vi "Read Voltage From Channel.vi"(8 "error in (no error)":errorcluster, 10 "Numeric":u8, 11 "IConfigure MultiChannel Voltmeter in":refnum<class "IConfigure MultiChannel Voltmeter.lvclass">) -> (0 "error out":errorcluster, 2 "Voltage":dbl format="%#_g V", 3 "IConfigure MultiChannel Voltmeter out":refnum<class "IConfigure MultiChannel Voltmeter.lvclass">)   [LabVIEW 2023, in "HAL Interfaces.lvlib" / "IConfigure MultiChannel Voltmeter.lvclass"]
uses:
  IConfigure MultiChannel Voltmeter.lvclass
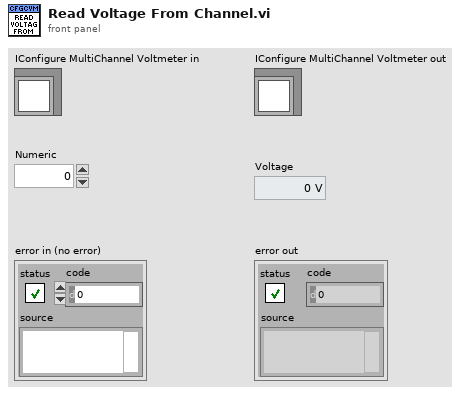
[diagram p1: front panel]
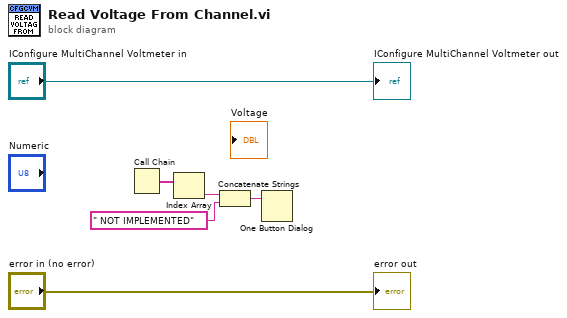
[diagram p0: block diagram]
diagram:
  n1 = Call Chain() -> (call chain=w4:string[])
  n2 = Index Array(array=w4) -> (element=w2:string)  [unwired: 1 in]
  n3 = Concatenate Strings(w2, " NOT IMPLEMENTED" ("string")) -> (w3:string)
  n4 = One Button Dialog(message=w3) -> ()  [unwired: 1 in, 1 out]
  "error out" <- "error in (no error)"
  "IConfigure MultiChannel Voltmeter out" <- "IConfigure MultiChannel Voltmeter in"
